vi "NOVO Peak Senzora.vi"() -> ()   [LabVIEW 2017]
uses:
  <vilib>/Waveform/WDTOps.llb/WDT Index Channel DBL.vi
panel:
  out "Izlaz":dbl[](array[numeric])
  out "Ulaz":dbl[](array[numeric])
  out "Round_Izlaz":dbl[](array[numeric])
  in  "Tab Control":enum32{"LIVE DATA", "Podesavanja"}(tab)
  out "Inteziteti ACC 1":waveform(dbl)(graph)
  out "Inteziteti ACC 2":waveform(dbl)(graph)
  out "Inteziteti ACC 3":waveform(dbl)(graph)
  out "TRENUTNI SIGNALI":dynamicdata(graph) caption="TRENUTNI SIGNALI !!!!"
  out "Iter":i32
  in  "File Name":string="TEST"
  in  "Ponavljanja":i32=20
  # "'Gore 1, Sredina 2, Dole 4, Miruje 8'"
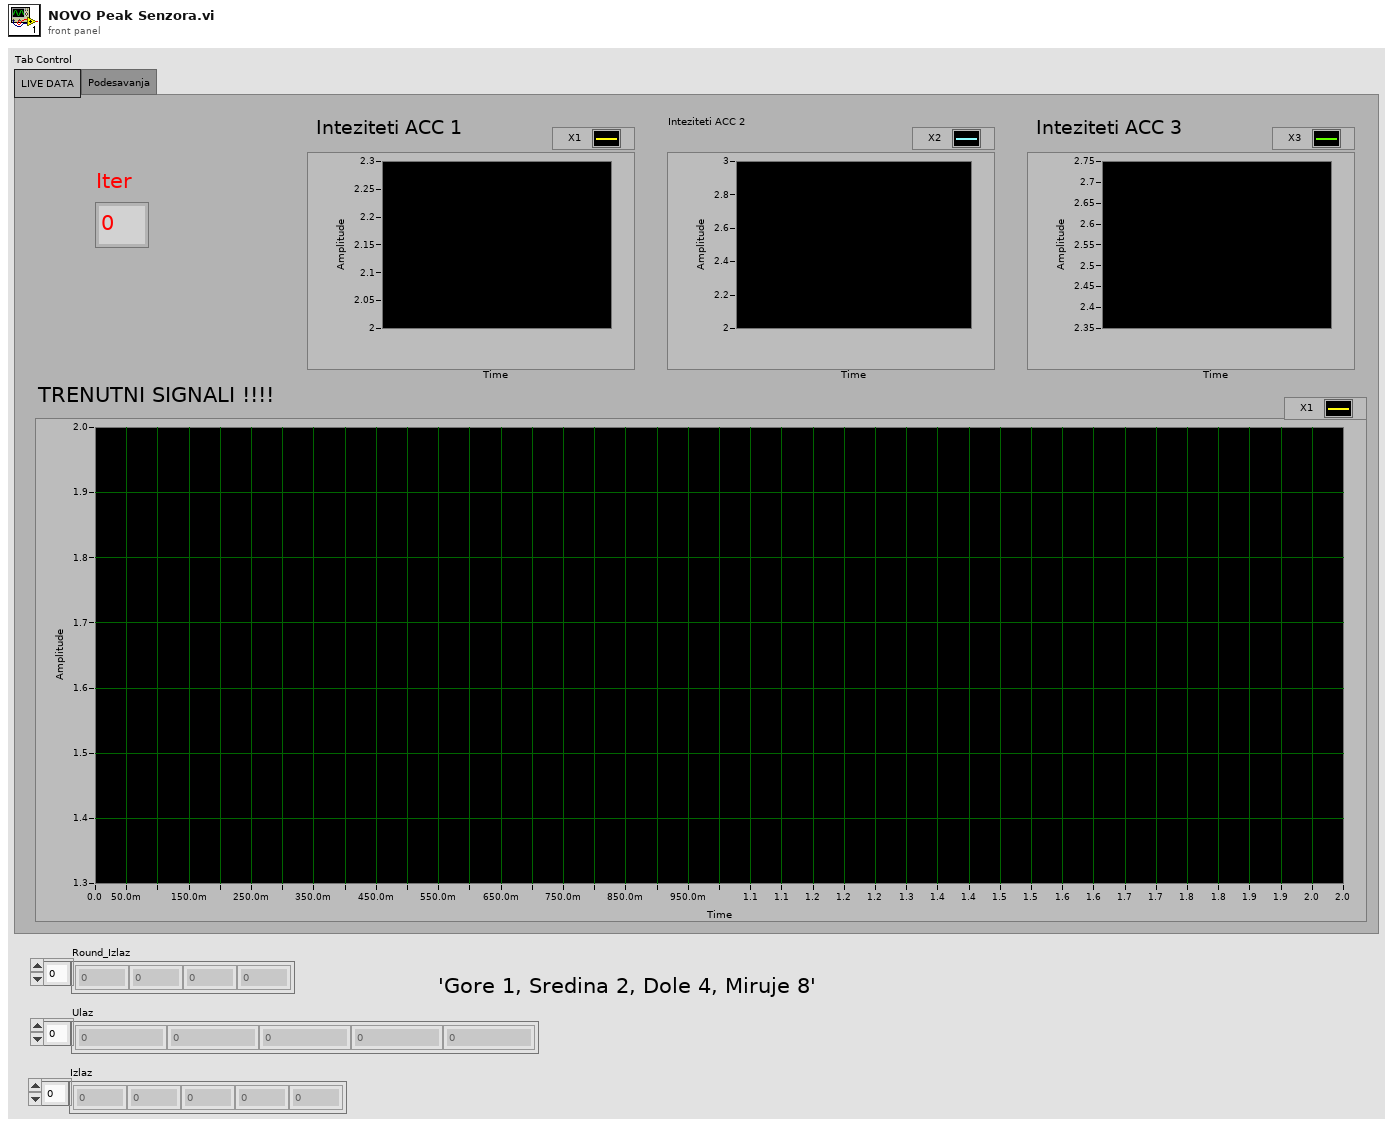
[diagram p1: front panel]
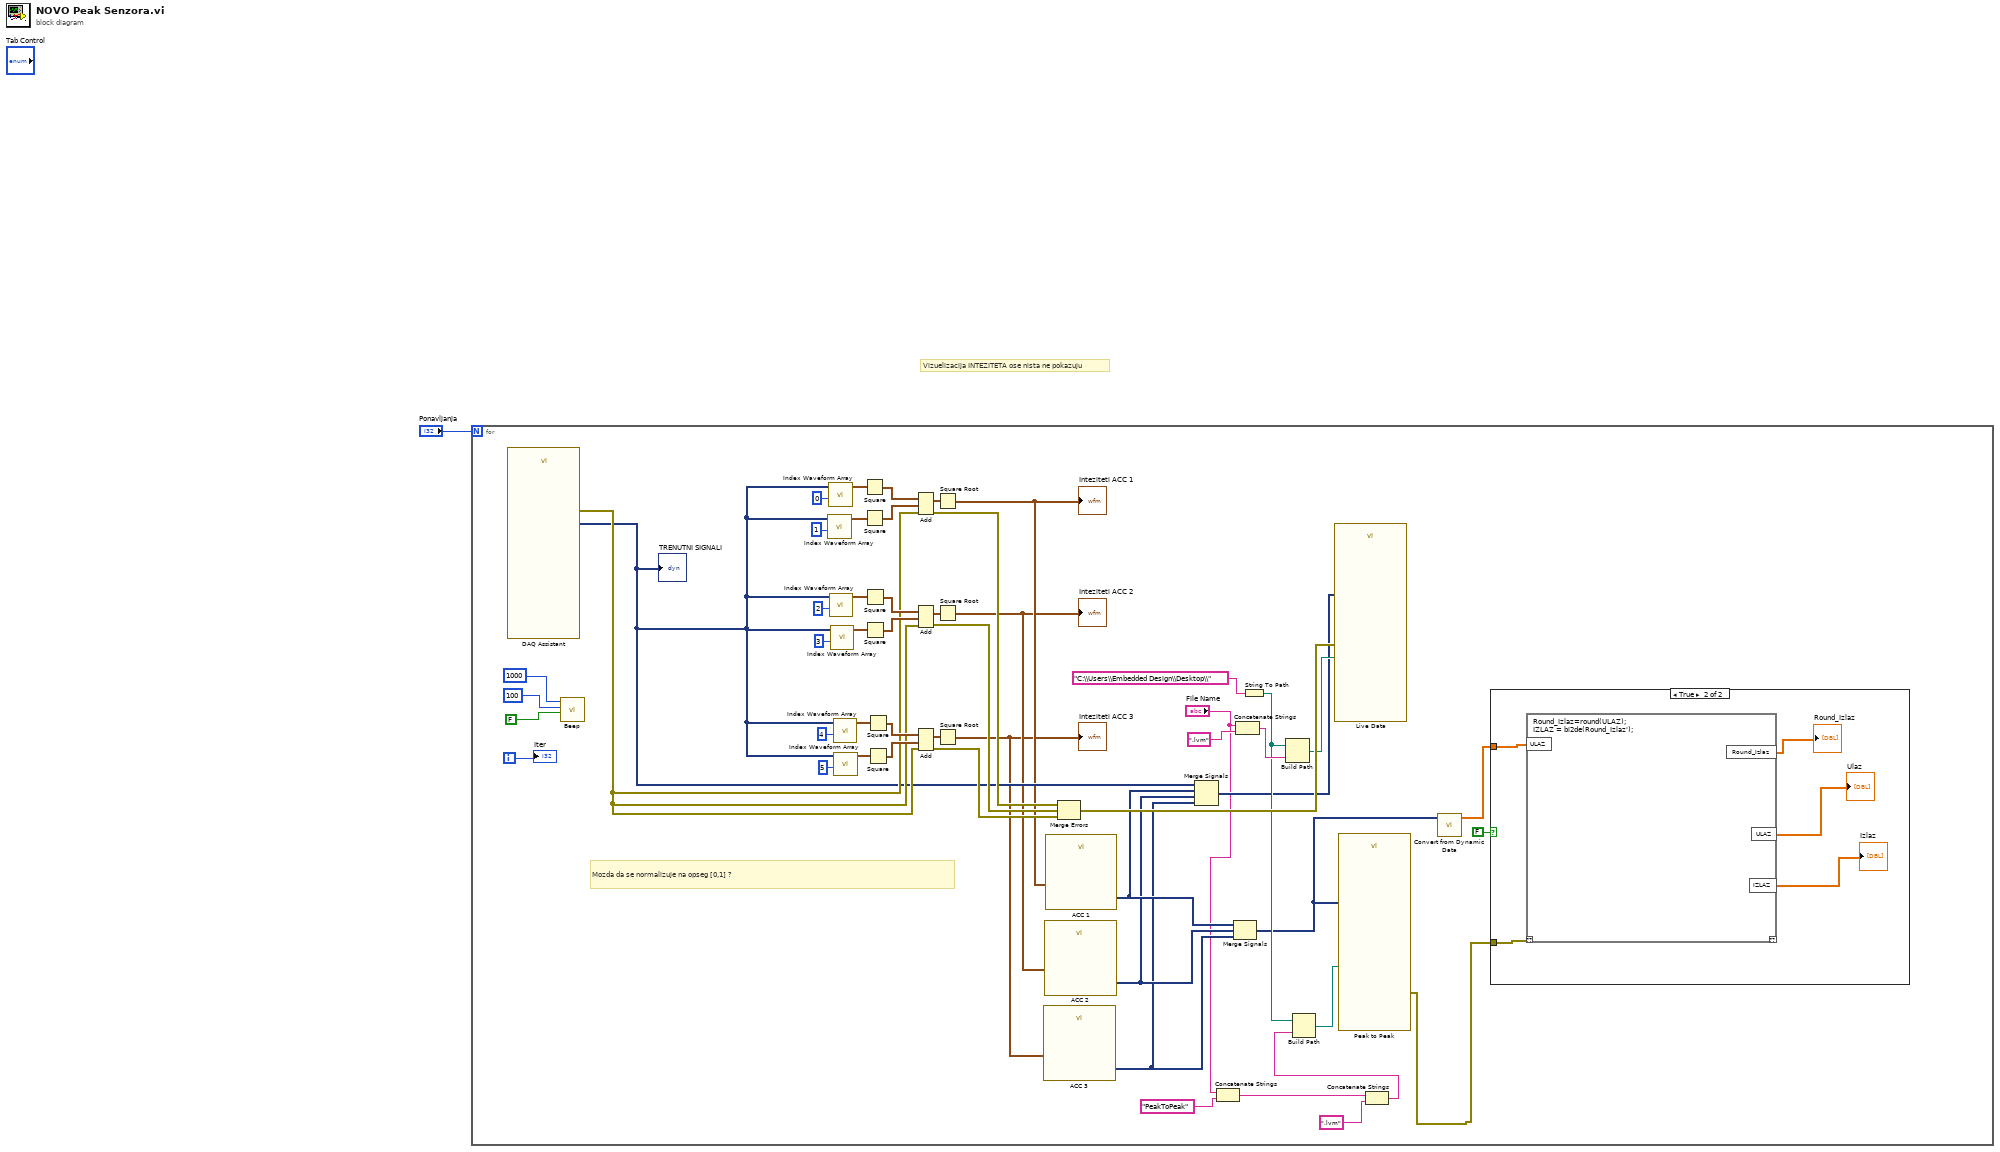
[diagram p0: block diagram]
diagram:
  # "Vizuelizacija INTEZITETA ose nista ne pokazuju"
  n1 = for {
    N: "Ponavljanja" -> [_]
    i -> [w21]
    # "Mozda da se normalizuje na opseg [0,1] ?"
    n2 = call "DAQ Assistant"() -> ("data"=w20:dynamicdata, "error out"=w25:errorcluster)  [unwired: 16 in, 2 out]
    "TRENUTNI SIGNALI" <- w20
    n3 = call <vilib>:"Beep.vi"("use system alert? (T)"=FALSE, "duration (msec)"=u32 100, "frequency (Hz)"=u32 1000) -> ()  [unwired: 9 in]
    n4 = call-poly <vilib>:"Index Waveform Array.vi"("index"=1, "waveform array"=w20) -> ("waveform"=w39:waveform(dbl))  [unwired: 8 in, 1 out]
    n5 = call-poly <vilib>:"Index Waveform Array.vi"("index"=0, "waveform array"=w20) -> ("waveform"=w40:waveform(dbl))  [unwired: 8 in, 1 out]
    n6 = call-poly <vilib>:"Index Waveform Array.vi"("index"=2, "waveform array"=w20) -> ("waveform"=w38:waveform(dbl))  [unwired: 8 in, 1 out]
    n7 = call-poly <vilib>:"Index Waveform Array.vi"("index"=3, "waveform array"=w20) -> ("waveform"=w37:waveform(dbl))  [unwired: 8 in, 1 out]
    n8 = call-poly <vilib>:"Index Waveform Array.vi"("index"=4, "waveform array"=w20) -> ("waveform"=w36:waveform(dbl))  [unwired: 8 in, 1 out]
    n9 = call-poly <vilib>:"Index Waveform Array.vi"("index"=5, "waveform array"=w20) -> ("waveform"=w35:waveform(dbl))  [unwired: 8 in, 1 out]
    n10 = Square(x=w40) -> (x^2=w34:waveform(dbl))
    n11 = Square(x=w39) -> (x^2=w33:waveform(dbl))
    n12 = Square(x=w38) -> (x^2=w32:waveform(dbl))
    n13 = Square(x=w37) -> (x^2=w31:waveform(dbl))
    n14 = Square(x=w36) -> (x^2=w30:waveform(dbl))
    n15 = Square(x=w35) -> (x^2=w29:waveform(dbl))
    n16 = Add(1:w33, 2:w34, 4:w25) -> (0:w28:waveform(dbl), 3:w24:errorcluster)
    n17 = Add(1:w31, 2:w32, 4:w25) -> (0:w27:waveform(dbl), 3:w23:errorcluster)
    n18 = Add(1:w29, 2:w30, 4:w25) -> (0:w26:waveform(dbl), 3:w22:errorcluster)
    n19 = Square Root(x=w28) -> (sqrt(x)=w16:waveform(dbl))
    "Inteziteti ACC 1" <- w16
    n20 = Square Root(x=w27) -> (sqrt(x)=w15:waveform(dbl))
    "Inteziteti ACC 2" <- w15
    n21 = Square Root(x=w26) -> (sqrt(x)=w14:waveform(dbl))
    "Inteziteti ACC 3" <- w14
    n22 = call "ACC 3"("Signals"=w14) -> ("Peak to Peak"=w10:dynamicdata)  [unwired: 13 in, 1 out]
    n23 = call "ACC 2"("Signals"=w15) -> ("Peak to Peak"=w11:dynamicdata)  [unwired: 13 in, 1 out]
    n24 = call "ACC 1"("Signals"=w16) -> ("Peak to Peak"=w12:dynamicdata)  [unwired: 13 in, 1 out]
    n25 = Merge Errors(w24, w23, w22) -> (w51:errorcluster)
    n26 = Merge Signals(w20, w12, w11, w10) -> (w13:dynamicdata)
    n27 = Concatenate Strings("File Name", "PeakToPeak" ("File Name 2")) -> (w7:string)
    n28 = Merge Signals(w12, w11, w10) -> (w4:dynamicdata)
    n29 = Concatenate Strings("File Name", ".lvm" ("name or relative path")) -> (w47:string)
    n30 = String To Path(string="C:\\Users\\Embedded Design\\Desktop\\") -> (path=w17:path)
    n31 = Build Path(base path=w17, name or relative path=w47) -> (appended path=w50:path)
    n32 = call "Live Data"("Signals"=w13, "error in (no error)"=w51, "Filename"=w50) -> ()  [unwired: 14 in, 3 out]
    n33 = Concatenate Strings(w7, ".lvm" ("name or relative path")) -> (w19:string)
    n34 = Build Path(base path=w17, name or relative path=w19) -> (appended path=w18:path)
    n35 = call "Peak to Peak"("Signals"=w4, "Filename"=w18) -> ("error out"=w5:errorcluster)  [unwired: 15 in, 2 out]
    n36 = call "Convert from Dynamic Data"("Dynamic Data Type"=w4) -> ("Array"=w3:dbl[])  [unwired: 3 in]
    n37 = case shown="True" FALSE {
      tunnel: w5 -> [_ w59]
      tunnel: w3 -> [_ w58]
      frame False {
      }
      frame True {
        n38 = script code="Round_Izlaz=round(ULAZ);\nIZLAZ = bi2de(Round_Izlaz');"("??"=w59, "ULAZ"=w58) -> ("Round_Izlaz"=→"Round_Izlaz":dbl[], "ULAZ"=→"Ulaz":dbl[], "IZLAZ"=→"Izlaz":dbl[])  [unwired: 1 out]
      }
    }
    "Iter" <- w21
  }
